vi "RMSRXOR2in2out.vi"() -> ()   [LabVIEW 2018]
uses:
  <vilib>/DAQmx/read.llb/DAQmx Read (Analog DBL 1Chan 1Samp).vi
  <vilib>/MakerHub/LINX/Public/Peripherals/Digital/Digital Write N Chans.vi
  <vilib>/Analysis/5stat.llb/RMS (DBL).vi
  <vilib>/MakerHub/LINX/Private/Local IO/LinxDigitalWrite.vi
  <vilib>/MakerHub/LINX/Public/Utilities/Check Channel.vi
  <vilib>/MakerHub/LINX/Public/Utilities/Open Serial.vi
  <vilib>/MakerHub/LINX/Private/Utilties/Generate Error.vi
  <vilib>/DAQmx/create/channels.llb/DAQmx Create Channel (AI-Voltage-Basic).vi
  <vilib>/DAQmx/configure/timing.llb/DAQmx Timing (Sample Clock).vi
  <vilib>/DAQmx/miscellaneous.llb/DAQmx Fill In Error Info.vi
  <vilib>/express/express arith-compare/Formula/XNode/ExpressFormulaBlockNode.xnode
  C/Program Files (x86)/National Instruments/LabVIEW 2018/instr.lib/XP Power PLS600/XP Power PLS600.lvlib
  <vilib>/ptbypt/NI_PtbyPt.lvlib
  <vilib>/MakerHub/LINX/LMH-LINX.lvlib
  <vilib>/Analysis/NI_AALPro.lvlib
panel:
  out "Current output (mA)":dbl
  in  "Filename":path=path "C:/Users/mtree/Desktop/testing.xls"
  in  "Visual Check?":bool
  out "Target Decimal Output of\nLogic Block":u8=1
  in  "Decimal Input into\nLogic Block":u8=1
  out "I/V Initial":dbl format="%#_13g"
  out "I/V Current":dbl format="%#_13g"
  in  "stop 5":bool
  out "Counter":dbl format="%#_13g"
  out "Actual Binary\nOutput":bool[](array[boolean])
  out "Target binary output":bool[](array[boolean])
  out "Binary Inputs into\nLogic Block":bool[](array[boolean])
  out "Current (mA) level\nfor output pins":dbl[](array[numeric])
  in  "Controls":T1(tab)
  in  "ADC Sample Mode":i32(ring)=10123 items=["Finite Samples"=10178, "Continuous Samples"=10123, "Hardware Timed Single Point"=12522]
  in  "ADC Minimum Value":dbl=-10.0 format="%0.2f"
  in  "ADC Input Channel 2":tag="cDAQ2Mod3/ai0"
  in  "ADC Sampling Rate":dbl=10000.0 format="%0.2f"
  in  "Sample Length for ADC mean":i32=100
  in  "ADC Maximum Value":dbl=10.0 format="%0.2f"
  in  "Serial Port for Arduino":refnum<visa-resource-name>="N/A"
  in  "Arduino Digital Outputs":u8[](array[numeric])=[2, 3, 4, 5, 6]
  in  "Fixed Resistor":dbl=350.0
  in  "Delay to avoid\nsampling bad data":dbl=0.4 caption="Delay Time (s)"
  in  "Number of\nOutput pins -1":i32=2
  in  "Over Voltage\nProtection":dbl=300.0 format="%#_13g"
  in  "Power Supply VISA resource name":refnum<visa-resource-name>
  in  "Set Max Current for FP":dbl=0.25 format="%#_13g"
  in  "Set Voltage":dbl=3.3 format="%#_13g"
  in  "Tolerance Range (in decimal, not %)":dbl=0.15 format="%#_13g"
  out "Numerical\nInput Troubleshoot":u32
  in  "Visual Check for\nTroubleshooting":bool
  out "index":i32
  out "Current Threshold":dbl=1000.0 format="%#_13g"
  out "Most Erroneous\nPin Output":dbl format="%#_13g"
  out "Most Erroneous\nPin Index Number":i32
  out "MUX channel":i32
  out "Ending Time Stamp 2":timestamp
  out "Voltage Output":dbl(graph)
  out "Over Allowable\nVoltage":bool
  out "Current level":dbl format="%#_13g"
  out "Voltage level":dbl format="%#_13g"
  out "Beginning Time Stamp":timestamp
  in  "stop":bool
  out "Done Training":bool
  # "NOTE: Pin 0 is Pin 1\non the PCB"
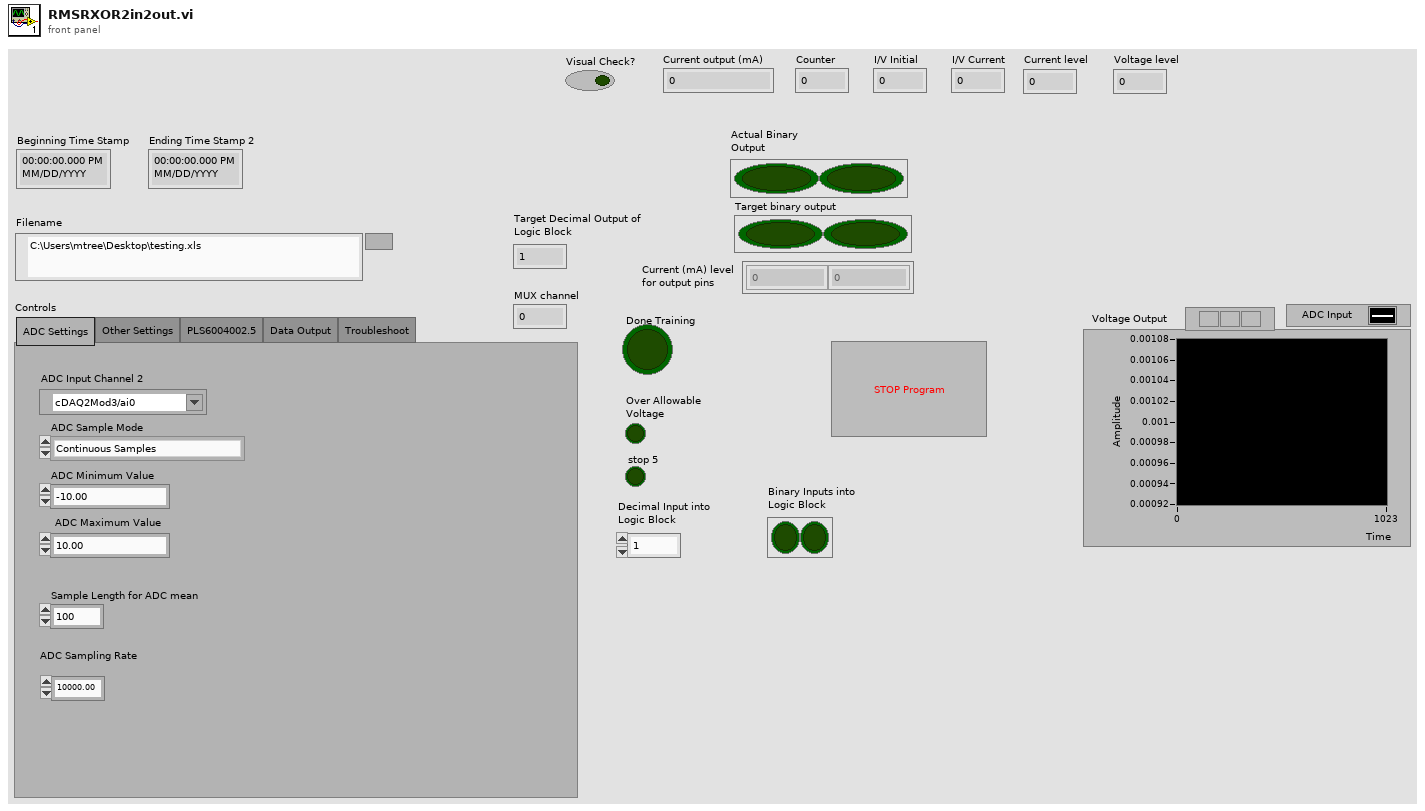
[diagram p1: front panel]
types:
  T1 = enum32{"ADC Settings", "Other Settings", "PLS6004002.5", "Data Output", "Troubleshoot"}
  T2 = cluster{"Baud Rate":u32, "Parity":u16, "Data Bits":u16, "Stop Bits":u16, "Flow Control":u16}
  T3 = typedef "LMH-LINX.lvlib/LINX Ref.ctl" = cluster{"IO":T4, "Interface":T5, "LINX Device Config":T6}
  T4 = typedef "LMH-LINX.lvlib/Platform.ctl" = enum16{"Remote", "Local"}
  T5 = typedef "LMH-LINX.lvlib/Interface.ctl" = enum16{"Serial", "TCP"}
  T6 = typedef "LMH-LINX.lvlib/Device.lvlib/LINX Device Config.ctl" = cluster{"Interface":T5, "COM Port":refnum<visa-resource-name>, "TCP Configuration":T7, "Device Family":u8, "Device ID":u8, "Device Name":string, "TCP Ref":refnum<k5>, "Channels":T8}
  T7 = typedef "LMH-LINX.lvlib/Device.lvlib/TCP Config.ctl" = cluster{"IP Address":string, "Port":u16}
  T8 = typedef "LMH-LINX.lvlib/Channels.ctl" = cluster{"DI":u8[], "DO":u8[], "AI":u8[], "AO":u8[], "PWM":u8[], "QE":u8[], "UART":u8[], "I2C 2":u8[], "SPI":u8[], "CAN":u8[], "Servo":u8[], "AI Ref (V)":dbl, "AI Resolution (Bits)":u8, "AO Ref (V)":dbl, "AO Resolution (Bits)":u8}
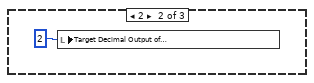
[diagram p2: hidden frame]
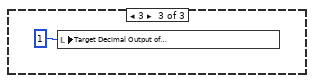
[diagram p3: hidden frame]
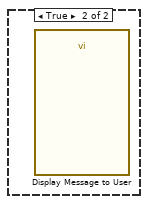
[diagram p5: hidden frame]
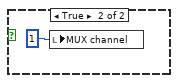
[diagram p6: hidden frame]
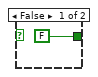
[diagram p9: hidden frame]
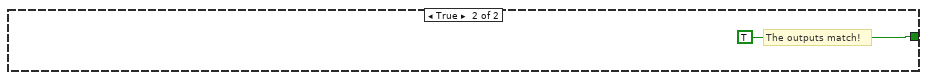
[diagram p11: hidden frame]
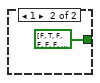
[diagram p13: hidden frame]
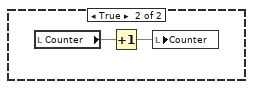
[diagram p15: hidden frame]
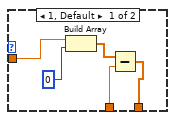
[diagram p16: hidden frame]
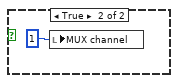
[diagram p19: hidden frame]
diagram:
  n1 = flat-sequence {
    tunnel: ["Arduino Digital Outputs"] -> w3
    tunnel: [w12] -> w2
    tunnel: [w11] -> w1
    tunnel: w3 -> [w381]
    tunnel: w2 -> [w380]
    tunnel: w1 -> [w379]
    frame #0 {
      n2 = while {
        stop <- w376 stop-if-true
        # "Event Structure is for universal stop of all while loops"
        n3 = event shown="[1] \"stop\": Mouse Up" {
          selector: _ -> [_ _]
          dyn-events: _ -> [_ _]
          timeout: _ -> [_ _]
          tunnel: [FALSE w378] -> w376
          event Timeout {
            n4 = event-data() -> ()  [unwired: 1 in, 3 out]
          }
          event "stop": Mouse Up {
            w378 = TRUE
            n5 = event-data() -> ()  [unwired: 1 in, 6 out]
            n6 = local write "stop"(w378) -> ()
          }
        }
      }
      n7 = flat-sequence {
        tunnel: [w297] -> w33
        tunnel: [w296] -> w32
        tunnel: [w327] -> w31
        tunnel: [w326] -> w30
        tunnel: ["Sample Length for ADC mean"] -> w29
        tunnel: [w316] -> w28
        tunnel: w33 -> [w316]
        tunnel: [w315] -> w27
        tunnel: w32 -> [w315]
        tunnel: w31 -> [w339]
        tunnel: w30 -> [w338]
        tunnel: w29 -> [w337]
        tunnel: [w336] -> w26
        tunnel: [w335] -> w25
        tunnel: [w331] -> w24
        tunnel: w28 -> [w333]
        tunnel: [w332] -> w23
        tunnel: w27 -> [w334]
        tunnel: w26 -> [w374]
        tunnel: w25 -> [w373]
        tunnel: w24 -> [w366]
        tunnel: w23 -> [w367]
        frame #0 {
          w303 = 2 items=["Minimum", "Maximum", "Value"]  # Voltage Setpoint Type
          w301 = TRUE  # Start XP power output
          w302 = 1 items=["Minimum", "Maximum", "Value"]  # Current Setpoint Type
          w300 = 1 items=["Local", "Remote", "Remote with Lock", "Voltage", "Current", "Dual"]  # System Mode
          w298 = TRUE  # Reset
          # "Configure Power Supply"
          # "Configure OVP, OCP, and OPP"
          # "Create the master stop"
          n8 = local write "Set Voltage"(3.3) -> ()
          n9 = call <instrlib>:"Initialize.vi"("Serial Configuration"=T2 {"Baud Rate"=57600, "Parity"=0, "Data Bits"=8, "Stop Bits"=10, "Flow Control"=0}, "Reset (True)"=w298, "VISA resource name"="Power Supply VISA resource name") -> ("error out"=w304:errorcluster, "VISA resource name out"=w305:refnum<visa-resource-name>)  [unwired: 7 in]
          n10 = call <instrlib>:"Configure System Mode.vi"("error in (no error)"=w304, "System Mode (0: Local)"=w300, "VISA resource name"=w305) -> ("error out"=w314:errorcluster, "VISA resource name out"=w313:refnum<visa-resource-name>)  [unwired: 7 in]
          n11 = call <instrlib>:"Configure Current Setpoint.vi"("error in (no error)"=w314, "Current Setpoint (0 amperes)"="Set Max Current for FP", "Current Setpoint Type (0: Minimum)"=w302, "VISA resource name"=w313) -> ("error out"=w311:errorcluster, "VISA resource name out"=w312:refnum<visa-resource-name>)  [unwired: 6 in]
          n12 = call "Configure Voltage Setpoint.vi"("error in (no error)"=w311, "Voltage Setpoint (0 volts)"="Set Voltage", "Voltage Setpoint Type (0: Minimum)"=w303, "VISA resource name"=w312) -> ("error out"=w310:errorcluster, "VISA resource name out"=w309:refnum<visa-resource-name>)  [unwired: 6 in]
          n13 = call "Set Output State.vi"("error in (no error)"=w310, "Output State (F: Disable)"=w301, "VISA resource name"=w309) -> ("error out"=w296:errorcluster, "VISA resource name out"=w297:refnum<visa-resource-name>)  [unwired: 7 in]
          "Done Training" <- FALSE ("Done Training")
        }
        frame #1 {
          # "Initialize the stop as false\nto reset the button from\nthe previous run."
          n14 = Get Date/Time In Seconds() -> (seconds since 1Jan1904=→"Beginning Time Stamp":timestamp)
          n15 = local write "stop"(FALSE) -> ()
          n16 = call-poly <vilib>:"DAQmx Create Virtual Channel.vi"("maximum value"="ADC Maximum Value", "minimum value"="ADC Minimum Value", "physical channels"="ADC Input Channel 2") -> ("task out"=w325:refnum<k21>, "error out"=w322:errorcluster)  [unwired: 11 in]
          n17 = call-poly <vilib>:"DAQmx Timing.vi"("task/channels in"=w325, "sample mode"="ADC Sample Mode", "rate"="ADC Sampling Rate", "error in"=w322) -> ("task out"=w324:refnum<k21>, "error out"=w323:errorcluster)  [unwired: 10 in]
          n18 = call <vilib>:"DAQmx Start Task.vi"("task/channels in"=w324, "error in"=w323) -> ("task out"=w327:refnum<k21>, "error out"=w326:errorcluster)  [unwired: 12 in]
        }
        frame #2 {
          n19 = while {
            tunnel: w339 -> [w363]
            tunnel: w338 -> [w362]
            tunnel: [w360] -> w336
            tunnel: [w359] -> w335
            tunnel: w337 -> [w358]
            stop <- w355 stop-if-true
            n20 = call-poly <vilib>:"DAQmx Read.vi"("task/channels in"=w363, "error in"=w362) -> ("task out"=w360:refnum<k21>, "data"=w361:dbl, "error out"=w359:errorcluster)  [unwired: 11 in]
            n21 = call <vilib>:"Mean PtByPt.vi"("x"=w361, "sample length"=w358) -> ("mean"=w354:dbl)  [unwired: 2 in, 1 out]
            "Voltage Output" <- w354
            n22 = Greater?(x="Over Voltage\nProtection", y=w354) -> (0:w357:bool)
            n23 = case shown="True" w357 {
              frame False {
                n24 = local write "Over Allowable\nVoltage"(TRUE ("Over Allowable\nVoltage")) -> ()
              }
              frame True {
                "Over Allowable\nVoltage" <- FALSE
              }
            }
            n25 = local read "stop"() -> (w355:bool)
          }
          n26 = while {
            shift-right: [w349] -> w332
            shift-left: w334 -> [w343]
            shift-right: [w348] -> w331
            shift-left: w333 -> [w341]
            stop <- w347 stop-if-true
            w351 = 2 items=["Minimum", "Maximum", "Value"]  # Voltage Setpoint Type
            n27 = call "Read Output.vi"("error in (no error)"=w343, "VISA resource name"=w341) -> ("error out"=w342:errorcluster, "Actual Current Level (amperes)"=→"Current level":dbl, "Actual Voltage Level (volts)"=→"Voltage level":dbl, "VISA resource name out"=w340:refnum<visa-resource-name>)  [unwired: 6 in]
            n28 = property on="Set Voltage" class="DigNum (strict)"() -> ("Value"=w346:dbl)  [unwired: 2 in, 2 out]
            n29 = call "Configure Voltage Setpoint.vi"("error in (no error)"=w342, "Voltage Setpoint (0 volts)"=w346, "Voltage Setpoint Type (0: Minimum)"=w351, "VISA resource name"=w340) -> ("error out"=w352:errorcluster, "VISA resource name out"=w353:refnum<visa-resource-name>)  [unwired: 6 in]
            n30 = call "Set Output State.vi"("error in (no error)"=w352, "Output State (F: Disable)"=TRUE, "VISA resource name"=w353) -> ("error out"=w349:errorcluster, "VISA resource name out"=w348:refnum<visa-resource-name>)  [unwired: 7 in]
            n31 = local read "stop"() -> (w347:bool)
          }
        }
        frame #3 {
          w368 = FALSE  # Disable Output
          # "Shut Down Power Supply"
          n32 = Get Date/Time In Seconds() -> (seconds since 1Jan1904=→"Ending Time Stamp 2":timestamp)
          n33 = call <vilib>:"DAQmx Stop Task.vi"("task/channels in"=w374, "error in"=w373) -> ("error out"=w375:errorcluster)  [unwired: 12 in, 1 out]
          n34 = call <vilib>:"Simple Error Handler.vi"("error in (no error)"=w375) -> ()  [unwired: 4 in, 5 out]
          n35 = call "Set Output State.vi"("error in (no error)"=w367, "Output State (F: Disable)"=w368, "VISA resource name"=w366) -> ("error out"=w369:errorcluster, "VISA resource name out"=w371:refnum<visa-resource-name>)  [unwired: 7 in]
          n36 = call <instrlib>:"Close.vi"("error in (no error)"=w369, "VISA resource name"=w371) -> ("error out"=w370:errorcluster)  [unwired: 9 in]
          n37 = call <vilib>:"Simple Error Handler.vi"("error in (no error)"=w370) -> ()  [unwired: 4 in, 5 out]
        }
      }
      n38 = case shown="1, Default" "Decimal Input into\nLogic Block" {
        frame 1, Default {
          "Target Decimal Output of\nLogic Block" <- 2.0
        }
        frame 2 {
          n39 = local write "Target Decimal Output of\nLogic Block"(2) -> ()
        }
        frame 3 {
          n40 = local write "Target Decimal Output of\nLogic Block"(1) -> ()
        }
      }
      n41 = call-poly <vilib>:"Open.vi"("Serial Port"="Serial Port for Arduino") -> ("Error Out"=w17:errorcluster, "LINX Resource"=w16:T3)  [unwired: 8 in, 1 out]
      n42 = Number To Boolean Array(number="Decimal Input into\nLogic Block") -> (Boolean array=w15:bool[])
      n43 = flat-sequence {
        tunnel: "Delay to avoid\nsampling bad data" -> [w52]
        tunnel: w17 -> [w51]
        tunnel: w16 -> [w50]
        tunnel: "Arduino Digital Outputs" -> [w49]
        tunnel: [w46] -> w13
        tunnel: [w45] -> w14
        tunnel: w15 -> [w39]
        tunnel: [w38] -> w5
        tunnel: [w82] -> w6
        tunnel: w5 -> [w82]
        tunnel: [w95] -> w21
        tunnel: [w94] -> w7
        tunnel: w6 -> [w94]
        tunnel: w21 -> [w102]
        tunnel: [w98] -> w8
        tunnel: w7 -> [w98]
        tunnel: [w112] -> w20
        tunnel: [w111] -> w9
        tunnel: w8 -> [w111]
        tunnel: w20 -> [w139]
        tunnel: "Arduino Digital Outputs" -> [w137]
        tunnel: w14 -> [w131]
        tunnel: [w136] -> w12
        tunnel: w13 -> [w132]
        tunnel: [w135] -> w11
        tunnel: "Arduino Digital Outputs" -> [w133]
        tunnel: w9 -> [w134]
        frame #0 {
          w40 = 1000.0  # Current Threshold must be originally set high for the algorithm
          w43 = 2  # Turn all the  SSR Outs On
          w47 = bool[][] [[FALSE, FALSE, FALSE, FALSE, FALSE, FALSE, FALSE, FALSE, FALSE, FALSE, FALSE, FALSE, FALSE, FALSE, FALSE, FALSE], [FALSE, FALSE, FALSE, FALSE, FALSE, FALSE, FALSE, FALSE, FALSE, FALSE, FALSE, FALSE, FALSE, TRUE, FALSE, FALSE], [FALSE, FALSE, FALSE, FALSE, FALSE, FALSE, FALSE, FALSE, FALSE, FALSE, FALSE, FALSE, FALSE, FALSE, TRUE, FALSE], [FALSE, FALSE, FALSE, FALSE, FALSE, FALSE, FALSE, FALSE, FALSE, FALSE, FALSE, FALSE, FALSE, TRUE, TRUE, FALSE], [FALSE, FALSE, FALSE, FALSE, FALSE, FALSE, FALSE, FALSE, FALSE, FALSE, FALSE, FALSE, FALSE, FALSE, FALSE, TRUE], [FALSE, FALSE, FALSE, FALSE, FALSE, FALSE, FALSE, FALSE, FALSE, FALSE, FALSE, FALSE, FALSE, TRUE, FALSE, TRUE], [FALSE, FALSE, FALSE, FALSE, FALSE, FALSE, FALSE, FALSE, FALSE, FALSE, FALSE, FALSE, FALSE, FALSE, TRUE, TRUE], [FALSE, FALSE, FALSE, FALSE, FALSE, FALSE, FALSE, FALSE, FALSE, FALSE, FALSE, FALSE, FALSE, TRUE, TRUE, TRUE]]  # Reed Relays,                                          EN,MUX
          # "I am only training a single path for the current code"
          n44 = Insert Into Array(array=w39, index=w43, new element=TRUE ("new element/subarray")) -> (w41:bool[])
          n45 = Boolean Array To Number(Boolean array=w41) -> (number=→"Numerical\nInput Troubleshoot":u32)
          n46 = call-poly <vilib>:"Digital Write.vi"("Error In"=w51, "Values"=w41, "DO Channels"=w49, "LINX Resource"=w50) -> ("Error Out"=w46:errorcluster, "LINX Resource"=w45:T3)  [unwired: 6 in]
          n47 = for {
            N: 2 -> [_]
            tunnel: w52 -> [w53]
            tunnel: w47 -> [w55] mode=indexing
            tunnel: [w54] -> w48 mode=indexing
            tunnel: [w53] -> w38 mode=indexing
            n48 = flat-sequence {
              tunnel: w55 -> [w56]
              tunnel: w53 -> [w58]
              tunnel: [w62] -> w54
              frame #0 {
                n49 = call "DAQ I/O FP Set"("data"=w56) -> ()  [unwired: 17 in, 2 out]
              }
              frame #1 {
                n50 = local read "stop"() -> (w57:bool)
                n51 = case shown="False" w57 {
                  tunnel: w58 -> [w59 _]
                  frame False {
                    n52 = while {
                      tunnel: w59 -> [w61]
                      stop <- TRUE stop-if-true
                      n53 = call "Time Delay to avoid relay switch noise"("Delay Time (s)"=w61) -> ()  [unwired: 10 in, 1 out]
                    }
                  }
                  frame True {
                  }
                }
              }
              frame #2 {
                n54 = local read "Voltage Output"() -> (w64:dbl)
                n55 = xnode "Formula"("X1"=w64, "X2"="Fixed Resistor") -> ("Result"=w62:dbl)  [unwired: 1 in, 1 out]
                "Current output (mA)" <- w62
              }
              frame #3 {
                n56 = case shown="False" "Visual Check for\nTroubleshooting" {
                  frame False {
                  }
                  frame True {
                    n57 = call "Display Message to User"() -> ()  [unwired: 10 in, 2 out]
                  }
                }
              }
              frame #4 {
                n58 = local read "MUX channel"() -> (w77:i32)
                n59 = Greater?(x=w77, y=1) -> (0:w78:bool)
                n60 = case shown="False" w78 {
                  frame False {
                    n61 = local read "MUX channel"() -> (w80:i32)
                    n62 = Increment(x=w80) -> (x+1=w79:i32)
                    n63 = local write "MUX channel"(w79) -> ()
                  }
                  frame True {
                    n64 = local write "MUX channel"(1 ("MUX channel")) -> ()
                  }
                }
              }
            }
          }
          "Current (mA) level\nfor output pins" <- w48
          "Binary Inputs into\nLogic Block" <- w39
          "Current Threshold" <- w40
        }
        frame #1 {
          # "Calculate Threshold"
          n65 = for {
            N: "Number of\nOutput pins -1" -> [_]
            i -> [w85]
            n66 = local read "Target Decimal Output of\nLogic Block"() -> (w87:u8)
            n67 = Number To Boolean Array(number=w87) -> (Boolean array=w84:bool[])
            "Target binary output" <- w84
            n68 = Index Array(array=w84, index=w85) -> (element=w86:bool)
            n69 = case shown="True" w86 {
              tunnel: w85 -> [_ w92]
              frame False {
              }
              frame True {
                n70 = local read "Current (mA) level\nfor output pins"() -> (w90:dbl[])
                n71 = local read "Current Threshold"() -> (w88:dbl)
                n72 = Index Array(array=w90, index=w92) -> (element=w89:dbl)
                n73 = Less?(x=w89, y=w88) -> (x < y?=w91:bool)
                n74 = case shown="True" w91 {
                  tunnel: w92 -> [_ _]
                  tunnel: w89 -> [_ w93]
                  frame False {
                  }
                  frame True {
                    n75 = local write "Current Threshold"(w93) -> ()
                  }
                }
              }
            }
            "index" <- w85
          }
        }
        frame #2 {
          # "Adjust the Threshold"
          n76 = local read "Current Threshold"() -> (w96:dbl)
          n77 = Multiply(x=w96, y=0.95) -> (x*y=w95:dbl)
          n78 = local write "Current Threshold"(w95) -> ()
        }
        frame #3 {
          # "Convert Outputs into a binary number\nbased on the Threshold"
          n79 = local read "Number of\nOutput pins -1"() -> (w100:i32)
          n80 = for {
            N: w100 -> [_]
            tunnel: w102 -> [w105]
            tunnel: [w103] -> w101 mode=indexing
            i -> [w104]
            n81 = local read "Current (mA) level\nfor output pins"() -> (w107:dbl[])
            n82 = Index Array(array=w107, index=w104) -> (element=w106:dbl)
            n83 = Greater?(x=w106, y=w105) -> (0:w108:bool)
            n84 = case shown="True" w108 {
              tunnel: [FALSE TRUE] -> w103
              frame False {
              }
              frame True {
              }
            }
          }
          "Actual Binary\nOutput" <- w101
          "Most Erroneous\nPin Output" <- 0.0 ("Most Erroneous\nOutput Pin")
        }
        frame #4 {
          # "Check to see if the output is correct"
          # "Calculate error for each pin"
          n85 = local read "Number of\nOutput pins -1"() -> (w116:i32)
          n86 = local read "Current (mA) level\nfor output pins"() -> (w113:dbl[])
          n87 = local read "Actual Binary\nOutput"() -> (w114:bool[])
          n88 = local read "Target binary output"() -> (w115:bool[])
          n89 = for {
            N: w116 -> [_]
            tunnel: w115 -> [w121] mode=indexing
            tunnel: w114 -> [w120] mode=indexing
            tunnel: w113 -> [w119] mode=indexing
            tunnel: [w117] -> w112 mode=indexing
            i -> [w118]
            n90 = Not Exclusive Or(1:w121, 2:w120) -> (0:w122:bool)
            n91 = case shown="False" w122 {
              tunnel: w119 -> [w126 _]
              tunnel: w118 -> [w125 _]
              tunnel: [FALSE ("Ouputs Match") TRUE] -> w117
              frame False {
                # "Identify the output pin with the\nmost error (has the most current\noutput)."
                n92 = local read "Most Erroneous\nPin Output"() -> (w123:dbl)
                n93 = Greater?(x=w126, y=w123) -> (0:w127:bool)
                n94 = case shown="True" w127 {
                  tunnel: w126 -> [_ w128]
                  tunnel: w125 -> [_ w129]
                  frame False {
                  }
                  frame True {
                    n95 = local write "Most Erroneous\nPin Output"(w128) -> ()
                    "Most Erroneous\nPin Index Number" <- w129
                  }
                }
              }
              frame True {
                # "The outputs match!"
              }
            }
          }
        }
        frame #5 {
          # "If any of the actual\nbinary outputs do \nnot match we train\nthe chip"
          # "End program"
          n96 = And Array Elements(Boolean array=w139) -> (logical AND=w138:bool)
          n97 = case shown="False" w138 {
            tunnel: w137 -> [w148 _]
            tunnel: w131 -> [w147 w293]
            tunnel: [w146 w293] -> w136
            tunnel: w132 -> [w145 w292]
            tunnel: [w144 w292] -> w135
            tunnel: w131 -> [_ _]
            tunnel: w132 -> [_ _]
            tunnel: w133 -> [_ _]
            tunnel: w134 -> [_ _]
            tunnel: w134 -> [w143 _]
            tunnel: w133 -> [w142 _]
            tunnel: w132 -> [w141 _]
            tunnel: w131 -> [w140 _]
            frame False {
              # "Train"
              n98 = flat-sequence {
                tunnel: w148 -> [w153]
                tunnel: w147 -> [w152]
                tunnel: [w151] -> w146
                tunnel: w145 -> [w150]
                tunnel: [w149] -> w144
                tunnel: w143 -> [w232]
                tunnel: w142 -> [w231]
                tunnel: w141 -> [w230]
                tunnel: w140 -> [w229]
                frame #0 {
                  n99 = flat-sequence {
                    tunnel: w153 -> [w158]
                    tunnel: w152 -> [w157]
                    tunnel: [w156] -> w151
                    tunnel: w150 -> [w155]
                    tunnel: [w154] -> w149
                    frame #0 {
                      n100 = disable-structure shown="Enabled" {
                        disable-tunnel: w158 -> [w164 _]
                        disable-tunnel: w157 -> [w163 w167]
                        disable-tunnel: [w162 w167] -> w156
                        disable-tunnel: w155 -> [w161 w166]
                        disable-tunnel: [w160 w166] -> w154
                        frame Enabled {
                          w165 = bool[] [FALSE, FALSE, FALSE, FALSE, FALSE]  # Shut Down  Arduino Outputs
                          # "Open all relays"
                          n101 = call "DAQ I/O Reset"("data"=u32[] [0, 0]) -> ()  [unwired: 17 in, 2 out]
                          n102 = call-poly <vilib>:"Digital Write.vi"("Error In"=w161, "Values"=w165, "DO Channels"=w164, "LINX Resource"=w163) -> ("Error Out"=w160:errorcluster, "LINX Resource"=w162:T3)  [unwired: 6 in]
                        }
                        frame Disabled {
                        }
                      }
                    }
                    frame #1 {
                      # "Close the reed relays to\ntrain erroneous pin"
                      n103 = local read "Most Erroneous\nPin Index Number"() -> (w174:i32)
                      n104 = local read "Binary Inputs into\nLogic Block"() -> (w171:bool[])
                      n105 = case shown="0, Default" w174 {
                        tunnel: [bool[] [TRUE, FALSE, FALSE, FALSE, FALSE, FALSE, FALSE, FALSE] bool[] [FALSE, TRUE, FALSE, FALSE, FALSE, FALSE, FALSE, FALSE]] -> w172
                        frame 0, Default {
                        }
                        frame 1 {
                        }
                      }
                      n106 = Array Subset(array=w171, index=0, length=4) -> (w168:bool[])
                      n107 = Insert Into Array(array=w168, index=4, new element=w172) -> (w173:bool[])
                      n108 = call "DAQ Assistant"("data"=w173) -> ()  [unwired: 17 in, 2 out]
                    }
                  }
                }
                frame #1 {
                  n109 = flat-sequence {
                    frame #0 {
                      n110 = call "Time Delay"("Delay Time (s)"=15.0) -> ()  [unwired: 10 in, 1 out]
                    }
                    frame #1 {
                      n111 = local read "Current level"() -> (w181:dbl)
                      n112 = local read "Voltage level"() -> (w180:dbl)
                      n113 = Divide(x=w181, y=w180) -> (x/y=w182:dbl)
                      n114 = Absolute Value(x=w182) -> (abs(x)=→"I/V Initial":dbl)
                    }
                    frame #2 {
                      n115 = while {
                        stop <- w195 stop-if-true
                        # "I/V to compare in while loop"
                        # "Compare to see if I/V Current is in 15%\nrange of I/V initial"
                        n116 = local read "I/V Current"() -> (w194:dbl)
                        n117 = local read "I/V Initial"() -> (w193:dbl)
                        n118 = local read "I/V Initial"() -> (w191:dbl)
                        n119 = local read "Current level"() -> (w199:dbl)
                        n120 = Wait (ms)(milliseconds to wait=1000) -> ()  [unwired: 1 out]
                        n121 = Stop(stop? (T)="stop 5") -> ()
                        n122 = local read "Counter"() -> (w204:dbl)
                        n123 = Greater?(x=w194, y=w193) -> (0:w192:bool)
                        n124 = case shown="True" w192 {
                          frame False {
                          }
                          frame True {
                            n125 = local read "I/V Current"() -> (w207:dbl)
                            n126 = local write "Counter"(0.0) -> ()
                            n127 = local write "I/V Initial"(w207) -> ()
                          }
                        }
                        n128 = Greater Or Equal?(x=w204, y=20.0) -> (x >= y?=w196:bool)
                        n129 = Greater?(x=w199, y=0.25) -> (0:w197:bool)
                        n130 = Or(x=w197, y=w196) -> (x .or. y?=w195:bool)
                        n131 = local read "Current level"() -> (w201:dbl)
                        n132 = local read "Voltage level"() -> (w200:dbl)
                        n133 = Subtract(x=1, y="Tolerance Range (in decimal, not %)") -> (x-y=w189:dbl)
                        n134 = Multiply(x=w191, y=w189) -> (x*y=w187:dbl)
                        n135 = Divide(x=w201, y=w200) -> (x/y=w185:dbl)
                        "I/V Current" <- w185
                        n136 = Less Or Equal?(x=w185, y=w187) -> (x <= y?=w186:bool)
                        n137 = case shown="False" w186 {
                          frame False {
                            n138 = local read "Set Voltage"() -> (w211:dbl)
                            n139 = local write "Counter"(0.0) -> ()
                            n140 = Wait (ms)(milliseconds to wait=1000) -> ()  [unwired: 1 out]
                            n141 = Increment(x=w211) -> (x+1=w210:dbl)
                            n142 = local write "Set Voltage"(w210) -> ()
                          }
                          frame True {
                            n143 = local read "Counter"() -> (w212:dbl)
                            n144 = Increment(x=w212) -> (x+1=w213:dbl)
                            n145 = local write "Counter"(w213) -> ()
                          }
                        }
                      }
                      n146 = local write "Counter"(0.0) -> ()
                    }
                  }
                  "Counter" <- 0.0
                }
                frame #2 {
                  n147 = call "Display Message to User2"() -> ()  [unwired: 10 in, 2 out]
                  n148 = local write "Done Training"(TRUE) -> ()
                  n149 = local write "Set Voltage"(3.3) -> ()
                }
                frame #3 {
                  # "SSRs"
                  n150 = for {
                    N: 2 -> [_]
                    tunnel: w232 -> [w261] mode=indexing
                    tunnel: w231 -> [w255]
                    shift-right: [w257] -> w224
                    shift-left: w230 -> [w259]
                    shift-right: [w256] -> w223
                    shift-left: w229 -> [w258]
                    tunnel: [w254] -> w226 mode=indexing
                    tunnel: bool[][] [[TRUE, FALSE, FALSE, FALSE, TRUE], [FALSE, TRUE, FALSE, FALSE, TRUE], [FALSE, FALSE, TRUE, FALSE, TRUE], [FALSE, FALSE, FALSE, TRUE, TRUE], [TRUE, TRUE, FALSE, FALSE, TRUE], [FALSE, TRUE, TRUE, FALSE, TRUE], [FALSE, FALSE, TRUE, TRUE, TRUE]] ("Values") -> [w253] mode=indexing
                    w260 = bool[][] [[FALSE, FALSE, FALSE, FALSE, FALSE, FALSE, FALSE, FALSE, FALSE, FALSE, FALSE, FALSE, FALSE, FALSE, FALSE, FALSE], [FALSE, FALSE, FALSE, FALSE, FALSE, FALSE, FALSE, FALSE, FALSE, FALSE, FALSE, FALSE, FALSE, TRUE, FALSE, FALSE], [FALSE, FALSE, FALSE, FALSE, FALSE, FALSE, FALSE, FALSE, FALSE, FALSE, FALSE, FALSE, FALSE, FALSE, TRUE, FALSE], [FALSE, FALSE, FALSE, FALSE, FALSE, FALSE, FALSE, FALSE, FALSE, FALSE, FALSE, FALSE, FALSE, TRUE, TRUE, FALSE], [FALSE, FALSE, FALSE, FALSE, FALSE, FALSE, FALSE, FALSE, FALSE, FALSE, FALSE, FALSE, FALSE, FALSE, FALSE, TRUE], [FALSE, FALSE, FALSE, FALSE, FALSE, FALSE, FALSE, FALSE, FALSE, FALSE, FALSE, FALSE, FALSE, TRUE, FALSE, TRUE], [FALSE, FALSE, FALSE, FALSE, FALSE, FALSE, FALSE, FALSE, FALSE, FALSE, FALSE, FALSE, FALSE, FALSE, TRUE, TRUE], [FALSE, FALSE, FALSE, FALSE, FALSE, FALSE, FALSE, FALSE, FALSE, FALSE, FALSE, FALSE, FALSE, TRUE, TRUE, TRUE]]  # Reed Relays,                                          EN,MUX
                    n151 = call-poly <vilib>:"Digital Write.vi"("Error In"=w259, "Values"=w253, "DO Channels"=w255, "LINX Resource"=w258) -> ("Error Out"=w257:errorcluster, "LINX Resource"=w256:T3)  [unwired: 6 in]
                    n152 = for {
                      N: 2 -> [_]
                      tunnel: w261 -> [w264]
                      tunnel: w260 -> [w263] mode=indexing
                      tunnel: [w262] -> w254 mode=indexing
                      n153 = flat-sequence {
                        tunnel: w263 -> [w265]
                        tunnel: w264 -> [w267]
                        tunnel: [w271] -> w262
                        frame #0 {
                          n154 = call "DAQ Assistant"("data"=w265) -> ()  [unwired: 17 in, 2 out]
                        }
                        frame #1 {
                          n155 = local read "stop"() -> (w266:bool)
                          n156 = case shown="False" w266 {
                            tunnel: w267 -> [w268 _]
                            frame False {
                              n157 = while {
                                tunnel: w268 -> [w270]
                                stop <- TRUE stop-if-true
                                n158 = call "Time Delay"("Delay Time (s)"=w270) -> ()  [unwired: 10 in, 1 out]
                              }
                            }
                            frame True {
                            }
                          }
                        }
                        frame #2 {
                          n159 = local read "Voltage Output"() -> (w272:dbl)
                          n160 = local read "Fixed Resistor"() -> (w273:dbl)
                          n161 = xnode "Formula"("X1"=w272, "X2"=w273) -> ("Result"=w271:dbl)  [unwired: 1 in, 1 out]
                          n162 = local write "Current output (mA)"(w271) -> ()
                        }
                        frame #3 {
                          n163 = case shown="True" "Visual Check?" {
                            frame False {
                            }
                            frame True {
                              n164 = call "Display Message to User3"() -> ()  [unwired: 10 in, 2 out]
                            }
                          }
                        }
                        frame #4 {
                          n165 = local read "MUX channel"() -> (w286:i32)
                          n166 = Greater?(x=w286, y=1) -> (0:w287:bool)
                          n167 = case shown="False" w287 {
                            frame False {
                              n168 = local read "MUX channel"() -> (w289:i32)
                              n169 = Increment(x=w289) -> (x+1=w288:i32)
                              n170 = local write "MUX channel"(w288) -> ()
                            }
                            frame True {
                              n171 = local write "MUX channel"(1 ("MUX channel")) -> ()
                            }
                          }
                        }
                      }
                    }
                  }
                  n172 = call <instrlib>:"Close.vi"("Error In"=w224, "LINX Resource"=w223) -> ("Error Out"=w227:errorcluster)  [unwired: 9 in]
                  n173 = Reshape Array(w226, 2) -> (w218:dbl[])
                  n174 = call <vilib>:"Simple Error Handler.vi"("error in (no error)"=w227) -> ()  [unwired: 4 in, 5 out]
                  n175 = Add Array Elements(numeric array=w218) -> (sum=w219:dbl)
                  n176 = for {
                    N: 2 -> [_]
                    tunnel: w219 -> [w240]
                    tunnel: w218 -> [w239] mode=indexing
                    tunnel: [w233] -> w217 mode=concatenating
                    n177 = local read "Target Decimal Output of\nLogic Block"() -> (w241:u8)
                    n178 = case shown="2" w241 {
                      tunnel: w240 -> [w245 w251]
                      tunnel: w239 -> [w244 w249]
                      tunnel: [w242 w247] -> w236
                      frame 1, Default {
                        n179 = Build Array(w245, 0) -> (w243:dbl[])
                        n180 = Subtract(x=w243, y=w244) -> (x-y=w242:dbl[])
                      }
                      frame 2 {
                        n181 = Build Array(0, w251) -> (w248:dbl[])
                        n182 = Subtract(x=w248, y=w249) -> (x-y=w247:dbl[])
                      }
                    }
                    n183 = local read "Current (mA) level\nfor output pins"() -> (w238:dbl[])
                    n184 = Add Array Elements(numeric array=w238) -> (sum=w237:dbl)
                    n185 = Divide(x=w236, y=w237) -> (x/y=w235:dbl[])
                    n186 = Multiply(x=w235, y=100) -> (x*y=w233:dbl[])
                  }
                  n187 = call-poly <vilib>:"RMS.vi"("X"=w217) -> ("rms value"=w216:dbl)  [unwired: 1 out]
                  n188 = call "Write To Measurement File2"("Signals"=w216, "Filename"="Filename") -> ()  [unwired: 15 in, 3 out]
                }
                frame #4 {
                  n189 = local write "stop"(TRUE) -> ()
                }
              }
            }
            frame True {
            }
          }
        }
      }
      "MUX channel" <- 1 ("MUX channel")
    }
    frame #1 {
      w383 = bool[] [FALSE, FALSE, FALSE, FALSE, FALSE]  # Shut Down  Arduino Outputs
      w388 = FALSE  # Reset Stop Button
      n190 = local write "Done Training"(TRUE ("Done Training")) -> ()
      n191 = local write "stop"(w388) -> ()
      n192 = call "DAQ I/O Reset"("data"=u32[] [0, 0]) -> ()  [unwired: 17 in, 2 out]
      n193 = call-poly <vilib>:"Digital Write.vi"("Error In"=w379, "Values"=w383, "DO Channels"=w381, "LINX Resource"=w380) -> ("Error Out"=w384:errorcluster, "LINX Resource"=w385:T3)  [unwired: 6 in]
      n194 = call <instrlib>:"Close.vi"("Error In"=w384, "LINX Resource"=w385) -> ("Error Out"=w386:errorcluster)  [unwired: 9 in]
      n195 = call <vilib>:"Simple Error Handler.vi"("error in (no error)"=w386) -> ()  [unwired: 4 in, 5 out]
    }
  }
